vi "Close SubVI.vi"(11 "SHIFTER DATA":T1) -> ()   [LabVIEW 2013, in "main.lvlib"]
uses:
  main.lvlib
  Components/TypeDef - SHIFTER.ctl
  Components/Dependencies.llb/Exit Event Ref.ctl
  New Design/Controls/Reference Cluster.ctl
  Components/Dependencies.llb/TLB_Dependencies.lvlib
types:
  T1 = typedef "main.lvlib/TypeDef - SHIFTER.ctl" = cluster{"Exit Event":T2, "Terminate Error":errorcluster, "User Parameter Controls":refnum<vi>[], "User Parameters":cluster{"Name":string, "CPR Number":string, "Measuring Type ":string, "Measuring Technique":string, "Measuring Limb":string, "Operator":string, "Doctor":string, "Comment":string, "AdditionalInfo":string, "RightArm":string[][], "LeftArm":string[][], "PalpationRight":string, "PalpationLeft":string, "Puls":dbl, "Temp One":dbl, "Temp Two":dbl, "ActivityBox":bool}, "System Parameters":cluster{"Paper Running?":bool, "GraphSelection":bool, "Date":string, "Active Page":string}, "Data Acquisition":cluster{"Acquisition":bool, "DAQmx Task":refnum<k21>, "DAQmx Error":errorcluster, "Record number":dbl, "RecordPath":path, "AcqDataRef":refnum<vi>, "Duration":timestamp, "Queue":refnum<queue>, "Control?":bool, "RelativeRecordPath":path}, "Reference signal":cluster{"DAQmx  Task ":refnum<k21>, "Monitor":bool, "Events":dbl, "Time":timestamp, "NullEvents":dbl, "RefDataRef":refnum<vi>, "Queue":refnum<queue>}, "Data Process":cluster{"SubpanelRef":refnum<vi>, "ActiveItemTag":string, "Queue":refnum<queue>}, "System Parameter Controls":refnum<vi>[], "Database":cluster{"PatientdataRef":refnum<file>, "PatientdataPath":path, "Blue Pressure":dbl, "Red Pressure":dbl, "ActiveItemTag":string, "Height Adjustment":dbl, "BluePositionArray":dbl[][], "RedPositionArray":dbl[][], "JournalPath":path}, "MWL":cluster{"PatientID":string, "Name":string, "DICOM Info":path, "DICOM Variables":string[], "Worklist":string[][]}, "Control":cluster{"Queue":refnum<queue>, "SignalCluster":cluster{"Pump":bool, "Finger":bool, "Ankle":bool, "Fast Def":bool, "Slow Def":bool, "Init Cal":bool, "Table Pres":bool, "Table":bool}}, "PageMenu":cluster{"VI Reference":refnum<vi>, "Queue":refnum<queue>}, "Profile":cluster{"VI Reference":refnum<vi>, "Queue":refnum<queue>}, "Configuration":cluster{"VI Reference":refnum<vi>, "Queue":refnum<queue>}, "Acquisition":cluster{"VI Reference":refnum<vi>, "Queue":refnum<queue>}, "Data":cluster{"VI Reference":refnum<vi>, "Queue":refnum<queue>}, "Journal":cluster{"VI Reference":refnum<vi>, "Queue":refnum<queue>}, "cRef":T3, "Bluetooth":cluster{"Queue":refnum<queue>, "VI Reference":refnum<vi>}}
  T2 = typedef "main.lvlib/TLB_Dependencies.lvlib/Exit Event Ref.ctl" = refnum<user-event>
  T3 = typedef "main.lvlib/Reference Cluster.ctl" = cluster{"Menu":cluster{"References":cluster{"Stop Acq":refnum<vi>, "MenuExit":refnum<vi>, "MenuStartADC":refnum<vi>, "PersonalInfoString":refnum<vi>, "Profile":refnum<vi>, "Configuration":refnum<vi>, "Acquisition":refnum<vi>, "Data":refnum<vi>, "Journal":refnum<vi>}}, "Profile":cluster{"References":cluster{"Search Patient ID":refnum<vi>, "Name":refnum<vi>, "CommentStr":refnum<vi>, "Listbox Patient ID":refnum<vi>, "ListboxDoctor":refnum<vi>, "ListboxOperator":refnum<vi>, "HospitalName":refnum<vi>, "HospitalDepartment":refnum<vi>, "HospitalAddress":refnum<vi>, "EditHospInfo":refnum<vi>, "Add Patient ID Btn":refnum<vi>, "Query Worklist":refnum<vi>}}, "Configuration":cluster{"References":cluster{"ListboxMeasurementArea":refnum<vi>, "ListboxMeasurementTechnique":refnum<vi>, "ListboxMeasurementMeth":refnum<vi>, "ListboxRightSegmentNr":refnum<vi>, "ListboxLeftSegmentNr":refnum<vi>, "HeightAdjustmentInt":refnum<vi>, "PalpationRight":refnum<vi>, "PalpationLeft":refnum<vi>, "ActivityBox":refnum<vi>}, "New method":cluster{"AddNewMeasurementBtn":refnum<vi>, "Left Time Table":refnum<vi>, "Right Time Table":refnum<vi>}, "Old method":cluster{"LeftArmPressureTable":refnum<vi>, "RightArmPressureTable":refnum<vi>, "SaveArmPressureBtn":refnum<vi>, "Puls":refnum<vi>, "TempTwo":refnum<vi>, "TempOne":refnum<vi>}, "Method":string}, "Acquisition":cluster{"References":cluster{"SegmentAcqString":refnum<vi>, "RingActGraph":refnum<vi>}}, "Data":cluster{"References":cluster{"cmString":refnum<vi>, "AdjustedHeight":refnum<vi>, "Menu":refnum<vi>, "Tangent On/Off":refnum<vi>, "FilterControl":refnum<vi>}}, "Journal":cluster{"References":cluster{"ReportSelection":refnum<vi>, "Data":refnum<vi>, "GenerateReport":refnum<vi>, "Menu":refnum<vi>, "Send To PACS":refnum<vi>}}}
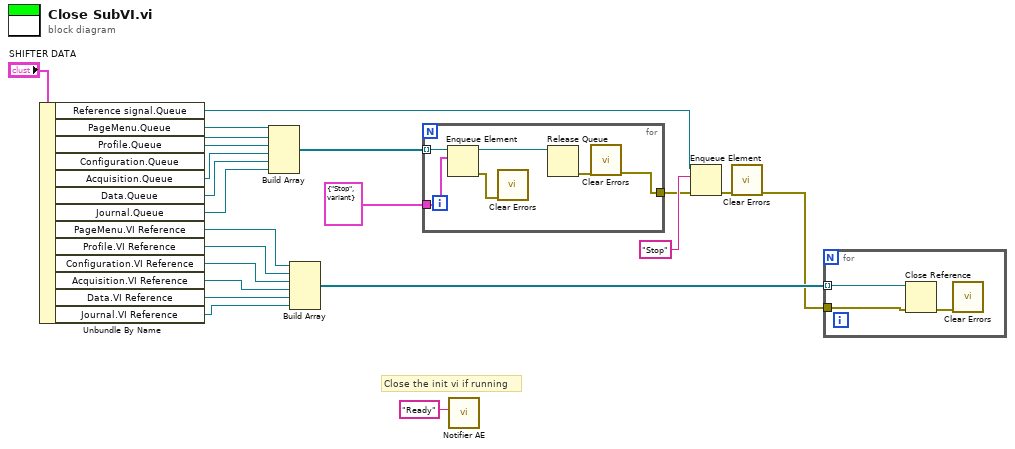
[diagram p0: block diagram]
diagram:
  # "Close the init vi if running"
  n1 = Unbundle By Name("SHIFTER DATA") -> ("Reference signal.Queue"=w5:refnum<queue>, "PageMenu.Queue"=w8:refnum<queue>, "Profile.Queue"=w9:refnum<queue>, "Configuration.Queue"=w10:refnum<queue>, "Acquisition.Queue"=w13:refnum<queue>, "Data.Queue"=w14:refnum<queue>, "Journal.Queue"=w15:refnum<queue>, "PageMenu.VI Reference"=w16:refnum<vi>, "Profile.VI Reference"=w17:refnum<vi>, "Configuration.VI Reference"=w18:refnum<vi>, "Acquisition.VI Reference"=w19:refnum<vi>, "Data.VI Reference"=w20:refnum<vi>, "Journal.VI Reference"=w21:refnum<vi>)
  n2 = Build Array(w8, w9, w10, w13, w14, w15) -> (w11:refnum<queue>[])
  n3 = Build Array(w16, w17, w18, w19, w20, w21) -> (w22:refnum<vi>[])
  n4 = for {
    tunnel: cluster{"Msg":string, "Data":variant} {"Msg"="Stop", "Data"=variant} ("element") -> [w28]
    tunnel: w11 -> [w27] mode=indexing
    tunnel: [w23] -> w2
    n5 = Enqueue Element(queue=w27, element=w28) -> (queue out=w25:refnum<queue>, error out=w26:errorcluster)  [unwired: 2 in, 1 out]
    n6 = call <vilib>:"Clear Errors.vi"("error in (no error)"=w26) -> ()  [unwired: 6 in, 1 out]
    n7 = Release Queue(queue=w25) -> (error out=w24:errorcluster)  [unwired: 2 in, 2 out]
    n8 = call <vilib>:"Clear Errors.vi"("error in (no error)"=w24) -> ("error out"=w23:errorcluster)  [unwired: 6 in]
  }
  n9 = call "Notifier AE.vi"("String"="Ready") -> ()  [unwired: 10 in, 1 out]
  n10 = Enqueue Element(queue=w5, element="Stop", error in (no error)=w2) -> (error out=w12:errorcluster)  [unwired: 1 in, 2 out]
  n11 = call <vilib>:"Clear Errors.vi"("error in (no error)"=w12) -> ("error out"=w3:errorcluster)  [unwired: 6 in]
  n12 = for {
    tunnel: w22 -> [w31] mode=indexing
    tunnel: w3 -> [w29]
    n13 = Close Reference(reference=w31, error in (no error)=w29) -> (error out=w30:errorcluster)
    n14 = call <vilib>:"Clear Errors.vi"("error in (no error)"=w30) -> ()  [unwired: 6 in, 1 out]
  }
